vi "DT9816_Multiplexer.vi"(0 "Sample Freq (Hz)":dbl=1000.0, 1 "Samples Per Channel":u32=100, 2 "Sample Mode":enum16{"Finite Samples", "Continuous Samples"}(ring)=enum."Continuous Samples", 3 "Multiplexer cycle freq. (Hz)":dbl=200.0, 6 "Number Chan to Read":u32=6, 8 "Channel list (Ain5 for channel volts)":string="0:4, 5", 9 "Vmax":dbl=10.0, 10 "Board Name":string="DT9816(00)", 11 "Vmin":dbl=-10.0, 12 "N banks":i32=8, 13 "Clock Duty Cycle (%)":dbl=50.0) -> (14 "2D volts out":dbl[][](array[numeric]), 15 "Multiplexer bank no.":i32[](array[numeric])=[5, 4, 4, 4, 5, 5, 4, 4, 4, 5, 5, 4, 4, 4, 5, 5, 4, 4, 4, 5, 5, 4, 4, 4, 5, 5, 4, 4, 4, 5, 5, 4, 4, 4, 5, 5, 4, 4, 4, 5, 5, 4, 4, 4, 5, 5, 4, 4, 4, 5, 5, 4, 4, 4, 5, 5, 4, 4, 4, 5, 5, 4, 4, 4, 5, 5, 4, 4, 4, 5, 5, 4, 4, 4, 5, 5, 4, 4, 4, 5, 5, 4, 4, 4, 5, 5, 4, 4, 4, 5, 5, 4, 4, 4, 5, 5, 4, 4, 4, 5], 17 "Actual Sample Freq":dbl, 18 "Data acq. final error":errorcluster, 19 "Clock error":errorcluster)   [LabVIEW 2013]
uses:
  <userlib>/LV-Link3/PolySubVIs/DtCreateCtrRateChan.vi
  <userlib>/LV-Link3/PolySubVIs/DtOLStartNormal.vi
  <userlib>/LV-Link3/PolySubVIs/DtCreateAinChan.vi
  <userlib>/LV-Link3/PolySubVIs/DtOLTimingSetInput.vi
  <userlib>/LV-Link3/PolySubVIs/DtOLReadMultiple2D.vi
panel:
  in  "V_DACmax":dbl=10.0
  # "N.B. Digital IO must be LAST on the channel list"
  # "Clock is output on CTR0 (pin17)"
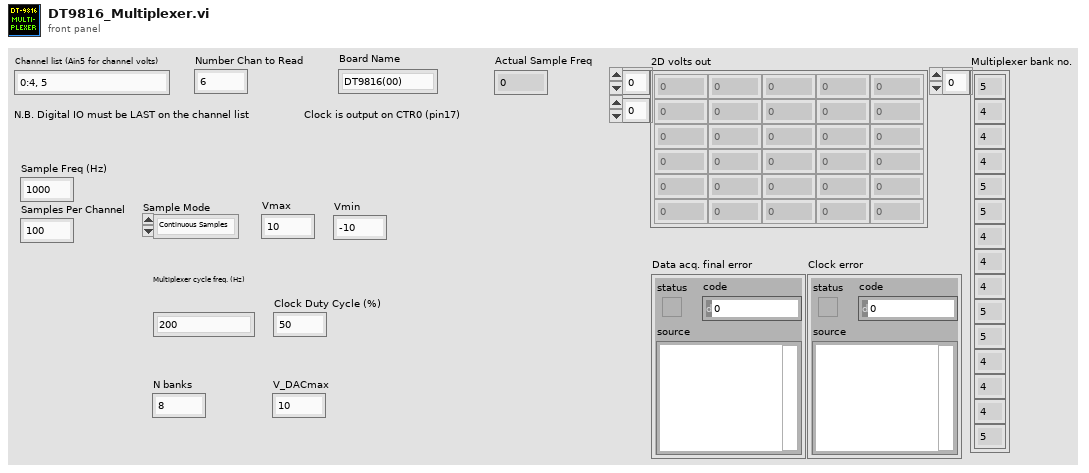
[diagram p1: front panel]
types:
  T1 = enum32{"Internal Clock", "External Clock", "No Timing"}
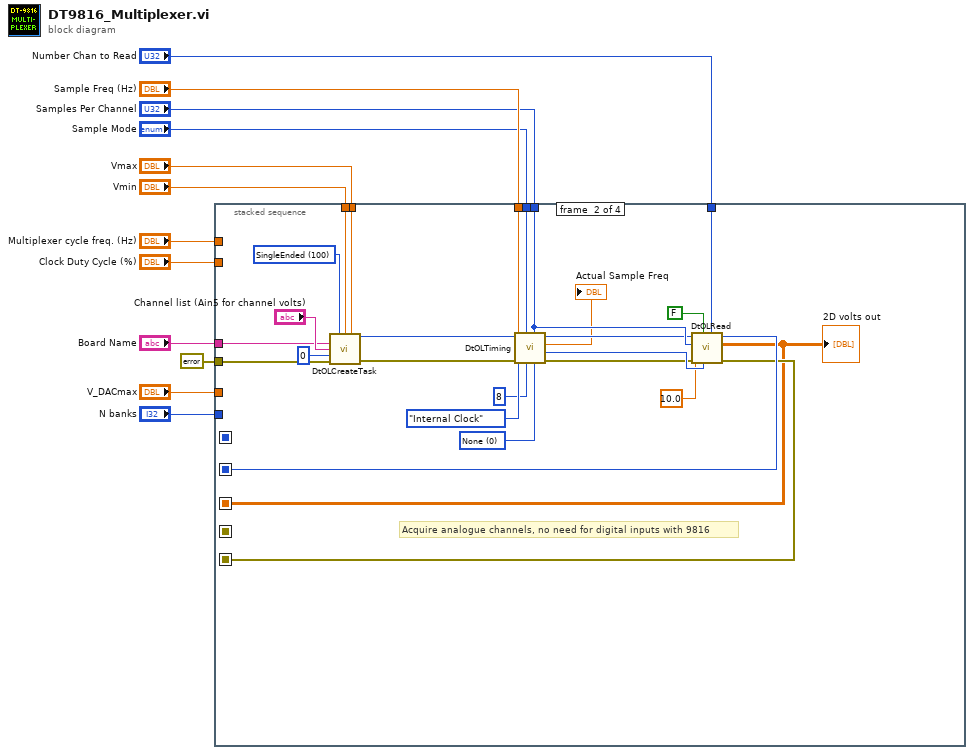
[diagram p0: block diagram]
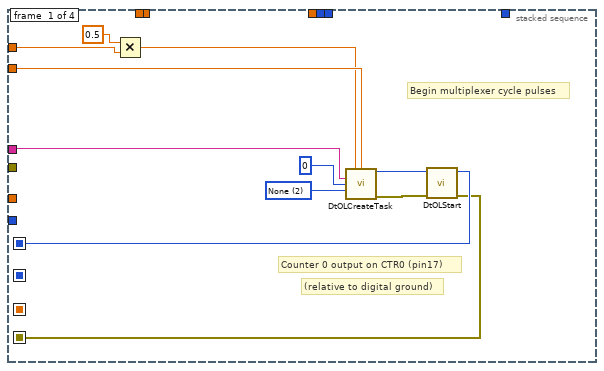
[diagram p2: hidden frame]
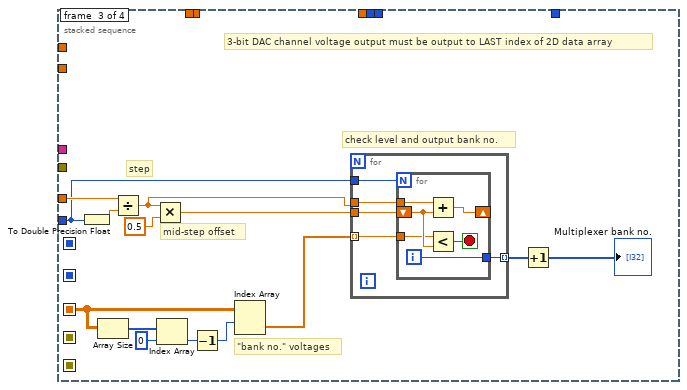
[diagram p3: hidden frame]
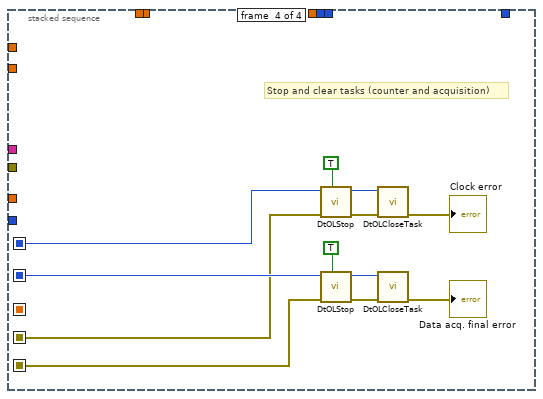
[diagram p4: hidden frame]
diagram:
  n1 = stacked-sequence {
    seq-local: [w18 _ _ _] -> [_ _ _ w75]
    seq-local: [_ w24 _ _] -> [_ _ w59 _]
    seq-local: [_ w27 _ _] -> [_ _ _ w80]
    seq-local: [_ w26 _ _] -> [_ _ _ w81]
    seq-local: [w17 _ _ _] -> [_ _ _ w74]
    tunnel: errorcluster {"status"=FALSE, "code"=0, "source"=""} ("error out") -> [_ w48 _ _]
    tunnel: "Sample Freq (Hz)" -> [_ w44 _ _]
    tunnel: "Sample Mode" -> [_ w41 _ _]
    tunnel: "Board Name" -> [w19 w38 _ _]
    tunnel: "Samples Per Channel" -> [_ w36 _ _]
    tunnel: "Number Chan to Read" -> [_ w33 _ _]
    tunnel: "Vmax" -> [_ w29 _ _]
    tunnel: "Vmin" -> [_ w28 _ _]
    tunnel: "Multiplexer cycle freq. (Hz)" -> [w15 _ _ _]
    tunnel: "Clock Duty Cycle (%)" -> [w16 _ _ _]
    tunnel: "V_DACmax" -> [_ _ w62 _]
    tunnel: "N banks" -> [_ _ w50 _]
    frame #0 {
      w22 = 2 items=["LowLevel", "HighLevel", "None"] ("Gate Type")
      # "Begin multiplexer cycle pulses"
      # "(relative to digital ground)"
      # "Counter 0 output on CTR0 (pin17)"
      n2 = Multiply(x=0.5, y=w15) -> (x*y=w13:dbl)
      n3 = call-poly <userlib>:"DtOLCreateTask.vi"("Requested\nFrequency (Hz)"=w13, "Duty Cycle"=w16, "Board Name"=w19, "Counter Num"=u32 0, "Gate Type"=w22) -> ("Task out"=w21:i32, "error out"=w20:errorcluster)  [unwired: 8 in, 1 out]
      n4 = call-poly <userlib>:"DtOLStart.vi"("error in (no error)"=w20, "Task in"=w21) -> ("error out"=w17:errorcluster, "Task out"=w18:i32)  [unwired: 8 in]
    }
    frame #1 {
      w39 = 0 items=["None", "Master", "Slave"] ("Sync Mode")
      w45 = 100 items=["SingleEnded"=100, "Differential"=101] ("Channel Type")
      # "Acquire analogue channels, no need for digital inputs with 9816"
      n5 = call-poly <userlib>:"DtOLCreateTask.vi"("Channel Type"=w45, "Range Min"=w28, "Range Max"=w29, "Board Name"=w38, "Channel"="Channel list (Ain5 for channel volts)", "Element"=u32 0, "error in (no error)"=w48) -> ("Task out"=w30:i32, "error out"=w42:errorcluster)  [unwired: 6 in, 1 out]
      n6 = call-poly <userlib>:"DtOLTiming.vi"("Sync Mode"=w39, "Samples Per Channel"=w36, "Num Buffers"=u32 8, "Sample Mode"=w41, "error in (no error)"=w42, "Timing"=T1."Internal Clock", "Sample Freq (Hz)"=w44, "Task in"=w30) -> ("error out"=w31:errorcluster, "Buffer Size"=w37:u32, "Actual Sample Freq"=→"Actual Sample Freq":dbl, "Task out"=w32:i32)
      n7 = call-poly <userlib>:"DtOLRead.vi"("Number Chan to Read"=w33, "Buffer size"=w37, "OnlyReadAvailable"=FALSE, "error in (no error)"=w31, "Timeout"=10.0, "Samples Per Channel"=w36, "Task in"=w32) -> ("error out"=w26:errorcluster, "2D Data out"=w24:dbl[][], "Task out"=w27:i32)  [unwired: 2 out]
      "2D volts out" <- w24
    }
    frame #2 {
      # "check level and output bank no."
      # "\"bank no.\" voltages"
      # "mid-step offset"
      # "step"
      # "3-bit DAC channel voltage output must be output to LAST index of 2D data array"
      n8 = To Double Precision Float(number=w50) -> (double precision float=w61:dbl)
      n9 = Array Size(array=w59) -> (size(s)=w57:i32[])
      n10 = Divide(x=w62, y=w61) -> (x/y=w52:dbl)
      n11 = Multiply(x=w52, y=0.5) -> (x*y=w54:dbl)
      n12 = Index Array(array=w57, index=0) -> (element=w56:i32)
      n13 = Decrement(x=w56) -> (x-1=w55:i32)
      n14 = Index Array(array=w59, index (row)=w55) -> (element=w53:dbl[])  [unwired: 1 in]
      n15 = for {
        tunnel: w53 -> [w65] mode=indexing
        tunnel: w54 -> [w67]
        tunnel: w52 -> [w66]
        tunnel: w50 -> [w64]
        tunnel: [w63] -> w51 mode=indexing
        n16 = for {
          N: w64 -> [_]
          shift-right: [w73] -> _
          shift-left: w67 -> [w71]
          tunnel: w66 -> [w72]
          tunnel: w65 -> [w70]
          tunnel: [w68] -> w63
          i -> [w68]
          stop <- w69 stop-if-true
          n17 = Add(x=w72, y=w71) -> (x+y=w73:dbl)
          n18 = Less?(x=w70, y=w71) -> (x < y?=w69:bool)
        }
      }
      n19 = Increment(x=w51) -> (x+1=→"Multiplexer bank no.":i32[])
    }
    frame #3 {
      # "Stop and clear tasks (counter and acquisition)"
      n20 = call <userlib>:"DtOLStop.vi"("Finish Buffer"=TRUE, "error in (no error)"=w74, "Task in"=w75) -> ("error out"=w78:errorcluster, "Task out"=w77:i32)  [unwired: 7 in]
      n21 = call <userlib>:"DtOLStop.vi"("Finish Buffer"=TRUE, "error in (no error)"=w81, "Task in"=w80) -> ("error out"=w83:errorcluster, "Task out"=w84:i32)  [unwired: 7 in]
      n22 = call <userlib>:"DtOLCloseTask.vi"("Error in"=w78, "Task in"=w77) -> ("Error Out"=→"Clock error":errorcluster)  [unwired: 9 in]
      n23 = call <userlib>:"DtOLCloseTask.vi"("Error in"=w83, "Task in"=w84) -> ("Error Out"=→"Data acq. final error":errorcluster)  [unwired: 9 in]
    }
  }
